vi "MGI Bezier Weights (SGL).vi"(1 "u":sgl format="%.2f") -> (0 "Bezier Weights":sgl[](array[numeric]) format="%.2f")   [LabVIEW 2016]
doc: "Computes an array of four weights, (1-u)^3, 3u(1-u)^2, 3u^2(1-u), and u^3 given u. u should be between 0 and 1.\n\nAuthored by David A. Moore\nsupport@mooregoodideas.com\nwww.mooregoodideas.com\n\nCopyright (c) 2010, Moore Good Ideas, Inc.\n\nAll rights reserved.\n\nRedistribution and use in source and binary forms, with or without modification, are permitted provided that the following conditions are met:\n\n * Redistributions of source code must retain the above copyright notice, this list of conditions and the following disclaimer.\n * Redistributions in binary form must reproduce the above copyright notice, this list of conditions and the following disclaimer in the documentation and/or other materials provided with the distribution.\n * Neither the name of Moore Good Ideas, Inc. nor the names of its contributors may be used to endorse or promote products derived from this software without specific prior written permission.\n\nTHIS SOFTWARE IS PROVIDED BY THE COPYRIGHT HOLDERS AND CONTRIBUTORS \"AS IS\" AND ANY EXPRESS OR IMPLIED WARRANTIES, INCLUDING, BUT NOT LIMITED TO, THE IMPLIED WARRANTIES OF MERCHANTABILITY AND FITNESS FOR A PARTICULAR PURPOSE ARE DISCLAIMED. IN NO EVENT SHALL THE COPYRIGHT OWNER OR CONTRIBUTORS BE LIABLE FOR ANY DIRECT, INDIRECT, INCIDENTAL, SPECIAL, EXEMPLARY, OR CONSEQUENTIAL DAMAGES (INCLUDING, BUT NOT LIMITED TO, PROCUREMENT OF SUBSTITUTE GOODS OR SERVICES; LOSS OF USE, DATA, OR PROFITS; OR BUSINESS INTERRUPTION) HOWEVER CAUSED AND ON ANY THEORY OF LIABILITY, WHETHER IN CONTRACT, STRICT LIABILITY, OR TORT (INCLUDING NEGLIGENCE OR OTHERWISE) ARISING IN ANY WAY OUT OF THE USE OF THIS SOFTWARE, EVEN IF ADVISED OF THE POSSIBILITY OF SUCH DAMAGE."
panel:
  # "(1-u)^3"
  # "3u*(1-u)^2"
  # "3u^2*(1-u)"
  # "u^3"
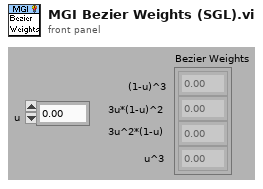
[diagram p1: front panel]
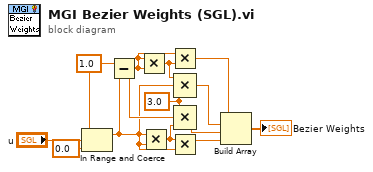
[diagram p0: block diagram]
diagram:
  w6 = sgl 3.0 ("Input")
  w2 = sgl 1.0 ("x")
  n1 = In Range and Coerce(upper limit=w2, x="u", lower limit=sgl 0.0) -> (coerced(x)=w3:sgl)  [unwired: 1 out]
  n2 = Subtract(x=w2, y=w3) -> (x-y=w9:sgl)
  n3 = Multiply(x=w9, y=w9) -> (x*y=w11:sgl)
  n4 = Multiply(x=w3, y=w3) -> (x*y=w10:sgl)
  n5 = Multiply(x=w9, y=w11) -> (x*y=w12:sgl)
  n6 = Multiply(x=w10, y=w3) -> (x*y=w13:sgl)
  n7 = Compound Arithmetic op=MULTIPLY(w11, w3, w6) -> (w7:sgl)
  n8 = Compound Arithmetic op=MULTIPLY(w6, w9, w10) -> (w8:sgl)
  n9 = Build Array(w12, w7, w8, w13) -> (→"Bezier Weights":sgl[])
